vi "Data Get Units.vi"(8 "error in (no error)":errorcluster, 11 "Data DVR in":refnum<data-value>) -> (0 "error out":errorcluster, 2 "Units DVR out":refnum<data-value>, 3 "Data DVR out":refnum<data-value>)   [LabVIEW 2010, in "MDSplus.lvlib"]
doc: "Return the units field. Return Empty if no units defined."
uses:
  <vilib>/MDSplus/Library/MDSplus.lvlib
  <vilib>/MDSplus/Classes/Data_Class/Data.lvclass
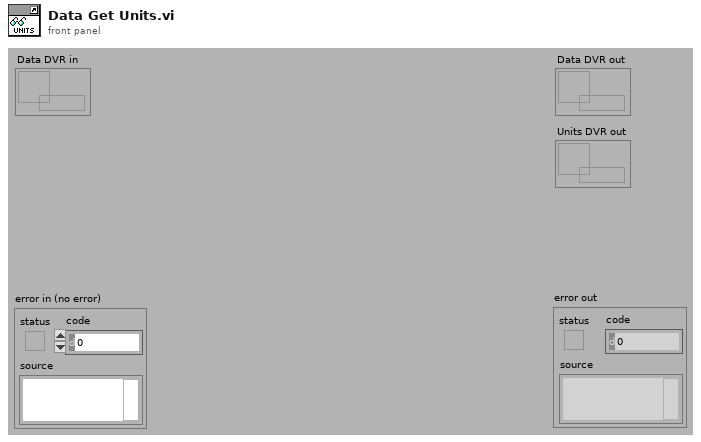
[diagram p1: front panel]
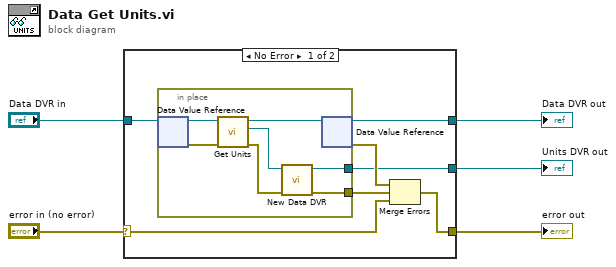
[diagram p0: block diagram]
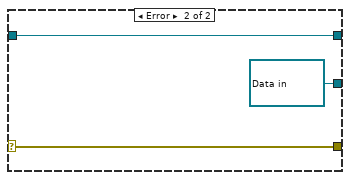
[diagram p2: hidden frame]
diagram:
  n1 = case shown="No Error" "error in (no error)" {
    selector: "error in (no error)" -> [w10 w22]
    tunnel: "Data DVR in" -> [w12 w21]
    tunnel: [w8 w22] -> w5
    tunnel: [w7 w21] -> w2
    tunnel: [w6 refnum<data-value> refnum ("Data DVR out")] -> w1
    frame No Error {
      n2 = in-place {
        in-place-border: [w13] -> w11
        in-place-border: [w15] -> w6
        n3 = in-place-dvr #1(w12) -> (w19:refnum<class "Data.lvclass">, w17:errorcluster)
        n4 = call-dynamic "Get Units.vi"("error in (no error)"=w17, "Data in"=w19) -> ("error out"=w14:errorcluster, "Units out"=w16:refnum<class "Data.lvclass">, "Data out"=w18:refnum<class "Data.lvclass">)  [unwired: 7 in]
        n5 = call <vilib>:"New Data DVR.vi"("error in (no error)"=w14, "Data in"=w16) -> ("error out"=w13:errorcluster, "Data DVR out"=w15:refnum<data-value>)  [unwired: 8 in]
        n6 = in-place-dvr #1(w18) -> (w7:refnum<data-value>, w9:errorcluster)
      }
      n7 = Merge Errors(w9, w11, w10) -> (w8:errorcluster)
    }
    frame Error {
    }
  }
  "error out" <- w5
  "Data DVR out" <- w2
  "Units DVR out" <- w1
